vi "Write Schema.vi"(8 "error in (no error)":errorcluster, 10 "Schema":string, 11 "Signal Analysis in":refnum<class "Signal Analysis.lvclass">) -> (0 "error out":errorcluster, 3 "Signal Analysis out":refnum<class "Signal Analysis.lvclass">)   [LabVIEW 2023, in "Data Analysis.lvlib" / "Signal Analysis.lvlib" / "Signal Analysis.lvclass"]
uses:
  Signal Analysis.lvclass
  Signal Analysis.lvclass/Signal Analysis.ctl
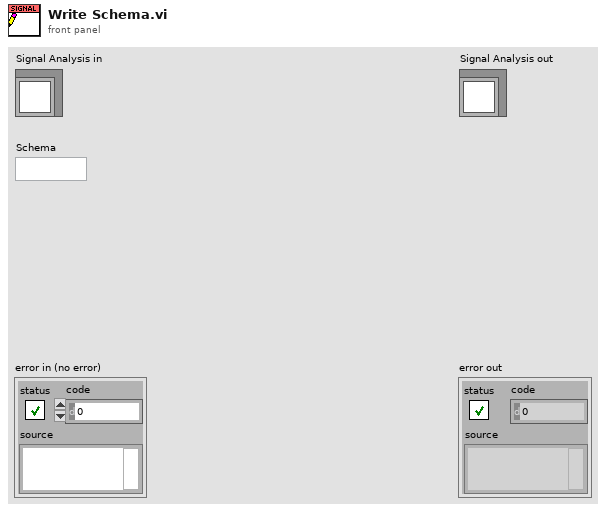
[diagram p1: front panel]
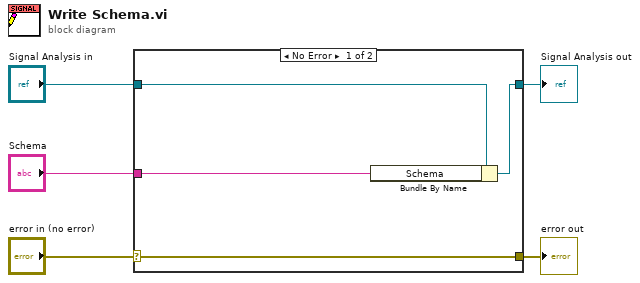
[diagram p0: block diagram]
diagram:
  n1 = case shown="No Error" "error in (no error)" {
    selector: "error in (no error)" -> [w9 w10]
    tunnel: [w9 w10] -> w4
    tunnel: [w7 w11] -> w2
    tunnel: "Signal Analysis in" -> [w8 w11]
    tunnel: "Schema" -> [w6 _]
    frame No Error {
      n2 = Bundle By Name(cluster=w8, "Schema"=w6) -> (w7:refnum<class "Signal Analysis.lvclass">)
    }
    frame Error {
    }
  }
  "error out" <- w4
  "Signal Analysis out" <- w2
